vi "RichToFlatni_bus_monitor_api_StopProcessReply.vi"(5 "OutputClusterType":T1, 11 "InputCluster":T3) -> (3 "OutputCluster":T1)   [LabVIEW 2025, in "bus_monitor_server.lvlib"]
uses:
  bus_monitor_server.lvlib
  ni_bus_monitor_api_StopProcessReply.ctl
  ni_bus_monitor_api_ErrorInfo.ctl
  ni_bus_monitor_api_StopProcessReply_Flat.ctl
  ni_bus_monitor_api_ErrorInfo_Flat.ctl
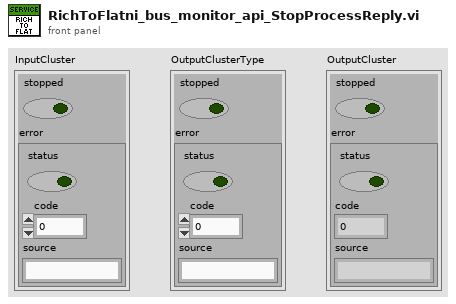
[diagram p1: front panel]
types:
  T1 = typedef "bus_monitor_server.lvlib/ni_bus_monitor_api_StopProcessReply_Flat.ctl" = cluster{"stopped":bool, "error":T2}
  T2 = typedef "bus_monitor_server.lvlib/ni_bus_monitor_api_ErrorInfo_Flat.ctl" = errorcluster
  T3 = typedef "bus_monitor_server.lvlib/ni_bus_monitor_api_StopProcessReply.ctl" = cluster{"stopped":bool, "error":T4}
  T4 = typedef "bus_monitor_server.lvlib/ni_bus_monitor_api_ErrorInfo.ctl" = errorcluster
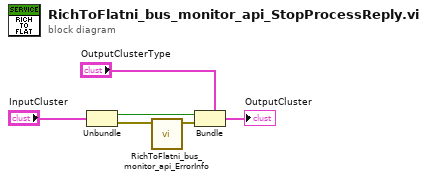
[diagram p0: block diagram]
diagram:
  n1 = Unbundle "Unbundle"("InputCluster") -> ("stopped"=w3:bool, "error"=w2:T4)
  n2 = call "RichToFlatni_bus_monitor_api_ErrorInfo.vi"("InputCluster"=w2) -> ("OutputCluster"=w1:T2)  [unwired: 10 in]
  n3 = Bundle "Bundle"(cluster="OutputClusterType", "stopped"=w3, "error"=w1) -> (→"OutputCluster":T1)
